vi "ZCAN_InitCAN(USBCANFD).vi"(0 "device_hande":u32, 5 "can_index":u32, 7 "ZCAN_InitCAN_Setting_USBCANFD":T1, 11 "error in (no error)":errorcluster caption="错误输入（无错误）") -> (8 "can_index_handle":u32, 15 "error out":errorcluster caption="错误输出")   [LabVIEW 2018]
doc: "设置CAN卡波特率，工作模式等。\n\n适用的设备：USBCANFD-100U、USBCANFD-200U、USBCANFD-MINI。"
uses:
  data_type/ZCAN_InitCAN_setting_USBCANFD.ctl
  bin/zlgcan_wrap.dll
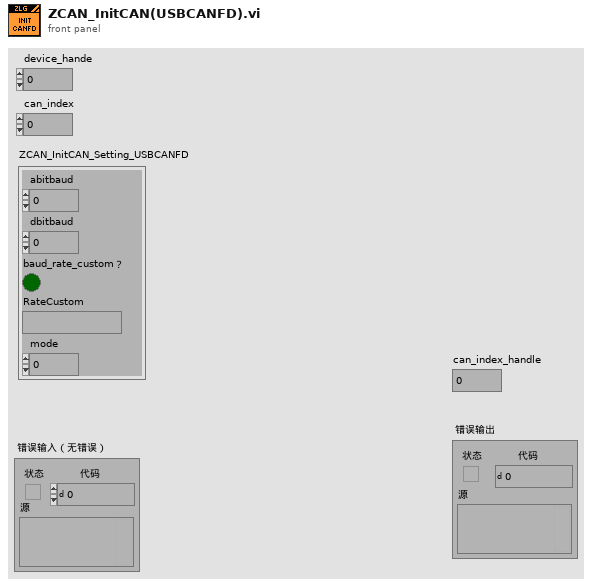
[diagram p1: front panel]
types:
  T1 = typedef "ZCAN_InitCAN_setting_USBCANFD.ctl" = cluster{"abitbaud":u32, "dbitbaud":u32, "baud_rate_custom？":bool, "RateCustom":string, "mode":u8}
  T2 = cluster{"can_type":u32, "can_type":u32, "can_type":u32, "can_type":u32, "can_type":u32, "can_type":u32, u8, "mode":u8, "pad":u16, "reserved":u32}
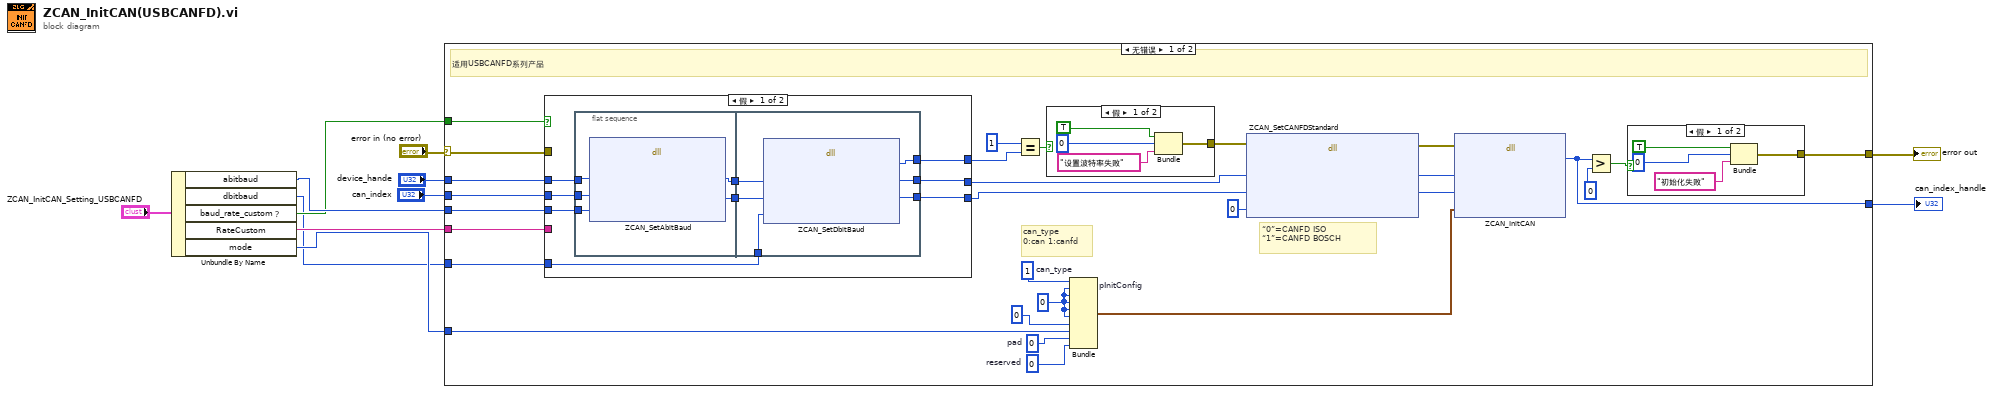
[diagram p0: block diagram]
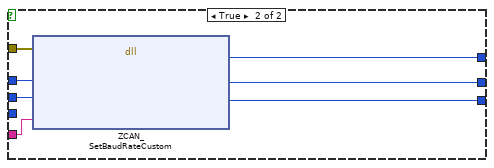
[diagram p4: hidden frame]
diagram:
  n1 = Unbundle By Name("ZCAN_InitCAN_Setting_USBCANFD") -> ("abitbaud"=w5:u32, "dbitbaud"=w1:u32, "baud_rate_custom？"=w4:bool, "RateCustom"=w3:string, "mode"=w2:u8)
  n2 = case shown="无错误" "error in (no error)" {
    selector: "error in (no error)" -> [w34 w75]
    tunnel: [w33 w75] -> w10
    tunnel: w4 -> [w39 _]
    tunnel: "device_hande" -> [w38 _]
    tunnel: "can_index" -> [w37 _]
    tunnel: w5 -> [w36 _]
    tunnel: w3 -> [w35 _]
    tunnel: w2 -> [w18 _]
    tunnel: [w32 _] -> w7
    tunnel: w1 -> [w12 _]
    frame No Error {
      w19 = u32 0  # reserved
      w20 = u16 0  # pad
      w17 = u32 0 ("can_type")
      w21 = u32 1  # can_type
      # "can_type\n0:can 1:canfd"
      # "“0”=CANFD ISO \n“1”=CANFD BOSCH"
      # "适用USBCANFD系列产品"
      n3 = case shown="假" w39 {
        tunnel: [w49 w74] -> w25
        tunnel: [w48 w73] -> w24
        tunnel: [w50 w72] -> w30
        tunnel: w38 -> [w56 w70]
        tunnel: w37 -> [w55 w69]
        tunnel: w36 -> [w54 _]
        tunnel: w35 -> [_ w71]
        tunnel: w34 -> [_ w68]
        tunnel: w12 -> [w51 _]
        frame False {
          n4 = flat-sequence {
            tunnel: w56 -> [w59]
            tunnel: w55 -> [w58]
            tunnel: w54 -> [w57]
            tunnel: [w61] -> w53
            tunnel: [w60] -> w52
            tunnel: w53 -> [w67]
            tunnel: w52 -> [w66]
            tunnel: w51 -> [w65]
            tunnel: [w64] -> w50
            tunnel: [w63] -> w49
            tunnel: [w62] -> w48
            frame #0 {
              n5 = dll-call lib="PTH2Fabs D\nUSBCANFD DEMO20200512USBCAN-I系列binzlgcan_wrap.dll" fn="ZCAN_SetAbitBaud" label="设置仲裁域波特率"("device_hande"=w59, "can_index"=w58, "abitbaud"=w57) -> ("device_hande"=w61:u32, "can_index"=w60:u32)  [unwired: 5 in, 2 out]
            }
            frame #1 {
              n6 = dll-call lib="PTH2Fabs D\nUSBCANFD DEMO20200512USBCAN-I系列binzlgcan_wrap.dll" fn="ZCAN_SetDbitBaud" label="设置数据域波特率"("device_hande"=w67, "can_index"=w66, "dbitbaud"=w65) -> ("return"=w64:u32, "device_hande"=w63:u32, "can_index"=w62:u32)  [unwired: 4 in, 2 out]
            }
          }
        }
        frame True {
          n7 = dll-call lib="PTH2Fabs D\nUSBCANFD DEMO20200512USBCAN-I系列binzlgcan_wrap.dll" fn="ZCAN_SetBaudRateCustom"(error in=w68, "device_handle"=w70, "can_index"=w69, "RateCustom"=w71) -> ("return"=w72:u32, "device_handle"=w74:u32, "can_index"=w73:u32)  [unwired: 3 in, 2 out]
        }
      }
      n8 = Equal?(x=1, y=w30) -> (x = y?=w29:bool)
      n9 = case shown="假" w29 {
        tunnel: [w44 _] -> w26
        frame False {
          n10 = Bundle("status"=TRUE, "code"=0, "消息"="设置波特率失败") -> (w44:cluster{"status":bool, "code":i32, "消息":string})  [unwired: 1 in]
        }
        frame True {
        }
      }
      n11 = Bundle "pInitConfig"("can_type"=w21, "can_type"=w17, "can_type"=w17, "can_type"=w17, "can_type"=w17, "can_type"=w17, u8 0, "mode"=w18, "pad"=w20, "reserved"=w19) -> (w15:T2)  [unwired: 1 in]
      n12 = dll-call lib="PTH2Fabs D\nUSBCANFD DEMO20200512USBCAN-I系列binzlgcan_wrap.dll" fn="ZCAN_SetCANFDStandard" ("ZCAN_InitCAN")(error in=w26, "device_handle"=w25, "can_index"=w24, "canfd_standard"=0) -> (error out=w22:errorcluster, "device_handle"=w14:u32, "can_index"=w13:i32)  [unwired: 4 in, 1 out]
      n13 = dll-call lib="PTH2Fabs D\nUSBCANFD DEMO20200512USBCAN-I系列binzlgcan_wrap.dll" fn="ZCAN_InitCAN"(error in=w22, "device_handle"=w14, "can_index"=w13, "pInitConfig"=w15) -> ("can_handle"=w32:u32)  [unwired: 5 in, 2 out]
      n14 = Greater?(x=w32, y=0) -> (0:w27:bool)
      n15 = case shown="假" w27 {
        tunnel: [w40 _] -> w33
        frame False {
          n16 = Bundle("status"=TRUE, "code"=0, "消息"="初始化失败") -> (w40:cluster{"status":bool, "code":i32, "消息":string})  [unwired: 1 in]
        }
        frame True {
        }
      }
    }
    frame Error {
    }
  }
  "error out" <- w10
  "can_index_handle" <- w7
